vi "Global_BeamBreaks.vi"() -> ()   [LabVIEW 2021]
panel:
  out "ConsumDetectors":bool[](array[boolean])
  in  "Beam breaks":bool[](array[boolean])
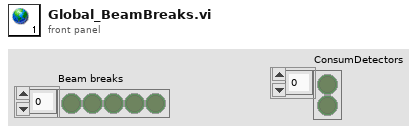
[diagram p1: front panel]
diagram:
